vi "GestionMenuGen.vi"(8 "error in":errorcluster caption="error out", 9 "ToDisableItems":string[](array[string]), 10 "ToEnableItems":string[](array[string]), 11 "référence de menu":refnum<k9>) -> (0 "error Out":errorcluster caption="error IO")   [LabVIEW 2010]
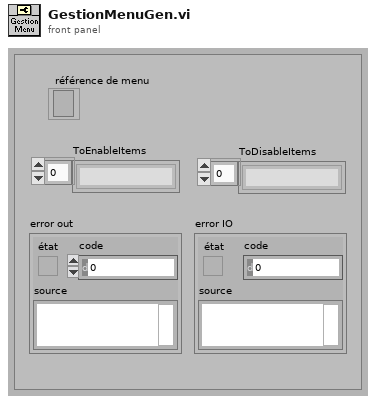
[diagram p1: front panel]
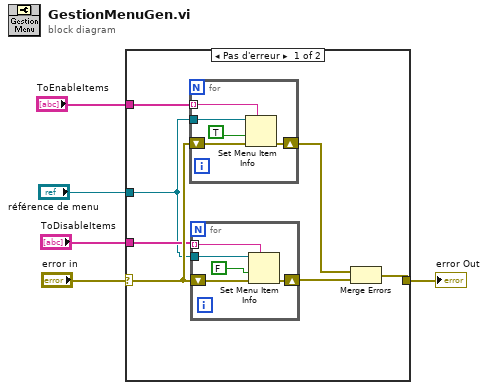
[diagram p0: block diagram]
diagram:
  n1 = case shown="Pas d'erreur" "error in" {
    selector: "error in" -> [w12 w23]
    tunnel: "référence de menu" -> [w6 _]
    tunnel: [w10 w23] -> w3
    tunnel: "ToDisableItems" -> [w8 _]
    tunnel: "ToEnableItems" -> [w7 _]
    frame No Error {
      n2 = for {
        tunnel: w7 -> [w22] mode=indexing
        tunnel: w6 -> [w21]
        shift-right: [w18] -> w9
        shift-left: w12 -> [w20]
        n3 = Set Menu Item Info(7:w22, 8:w20, 9:TRUE ("enabled"), 11:w21) -> (0:w18:errorcluster)  [unwired: 3 in, 1 out]
      }
      n4 = for {
        tunnel: w8 -> [w15] mode=indexing
        shift-right: [w16] -> w11
        shift-left: w12 -> [w17]
        tunnel: w6 -> [w13]
        n5 = Set Menu Item Info(7:w15, 8:w17, 9:FALSE ("enabled"), 11:w13) -> (0:w16:errorcluster)  [unwired: 3 in, 1 out]
      }
      n6 = Merge Errors(w9, w11) -> (w10:errorcluster)
    }
    frame Error {
    }
  }
  "error Out" <- w3
